vi "Spectrometer Digikröm.vi"(8 "error in (no error)":errorcluster, 11 "Spectrometer Digikröm in":refnum<class "Spectrometer Digikröm.lvclass">) -> (0 "error out":errorcluster, 3 "Spectrometer Digikröm out":refnum<class "Spectrometer Digikröm.lvclass">)   [LabVIEW 2009, in "Spectrometer Digikröm.lvclass"]
uses:
  Spectrometer Digikröm.lvclass
  Global/GPIB Numbers.vi
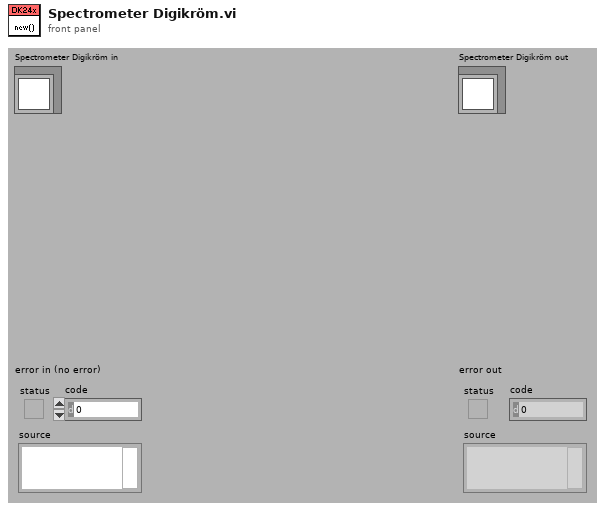
[diagram p1: front panel]
types:
  T1 = typedef "GPIB Type Def.ctl" = cluster{"Name":string, "bus":dbl, "GPIB":dbl, "GPIB as string":string, "byte":i32, "VISA Resource Name":refnum<visa-resource-name>}
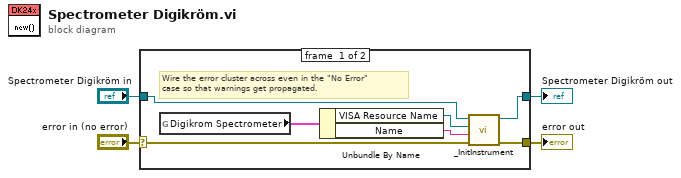
[diagram p0: block diagram]
diagram:
  n1 = case shown="No Error" "error in (no error)" {
    selector: "error in (no error)" -> [w6 w13]
    tunnel: [w5 w13] -> w3
    tunnel: [w10 w12] -> w1
    tunnel: "Spectrometer Digikröm in" -> [w11 w12]
    frame #0 {
      # "Wire the error cluster across even in the \"No Error\"\ncase so that warnings get propagated."
      n2 = global read "GPIB Numbers.vi" "Digikrom Spectrometer"() -> (w9:T1)
      n3 = Unbundle By Name(w9) -> ("VISA Resource Name"=w8:refnum<visa-resource-name>, "Name"=w7:string)
      n4 = call-dynamic "_InitInstrument.vi"("error in (no error)"=w6, "Name"=w7, "VISA Resource Name"=w8, "Instrument in"=w11) -> ("error out"=w5:errorcluster, "Instrument out"=w10:refnum<class "Spectrometer Digikröm.lvclass">)  [unwired: 2 in, 4 out]
    }
    frame #1 {
    }
  }
  "error out" <- w3
  "Spectrometer Digikröm out" <- w1
